vi "Check Loop Error.vi"(9 "Ignore Errors":i32[](array[numeric]) caption="忽略错误", 10 "error to process":errorcluster caption="待处理的错误", 11 "Message Queue":refnum<queue> caption="消息队列") -> (2 "Enqueued Error?":bool caption="错误入队列？", 3 "dup Message Queue":refnum<queue> caption="消息队列副本")   [LabVIEW 2013]
doc: "检查“处理的错误”，查看代码值是否与“忽略错误”数组中的任意值相匹配。如果是，则忽略。如果否，发送包含错误数据的错误信息至消息处理循环，以进行深入处理。"
uses:
  Message Queue/Message Cluster.ctl
  Message Queue/Enqueue Message (Single).vi
  Message Queue/Message Queue.lvlib
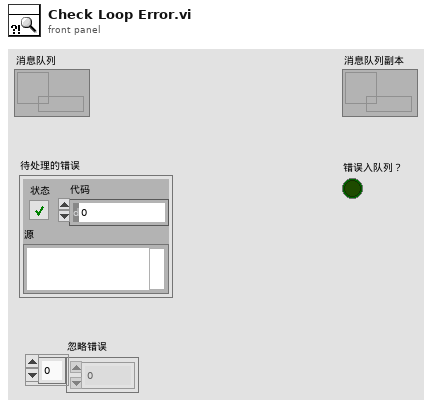
[diagram p1: front panel]
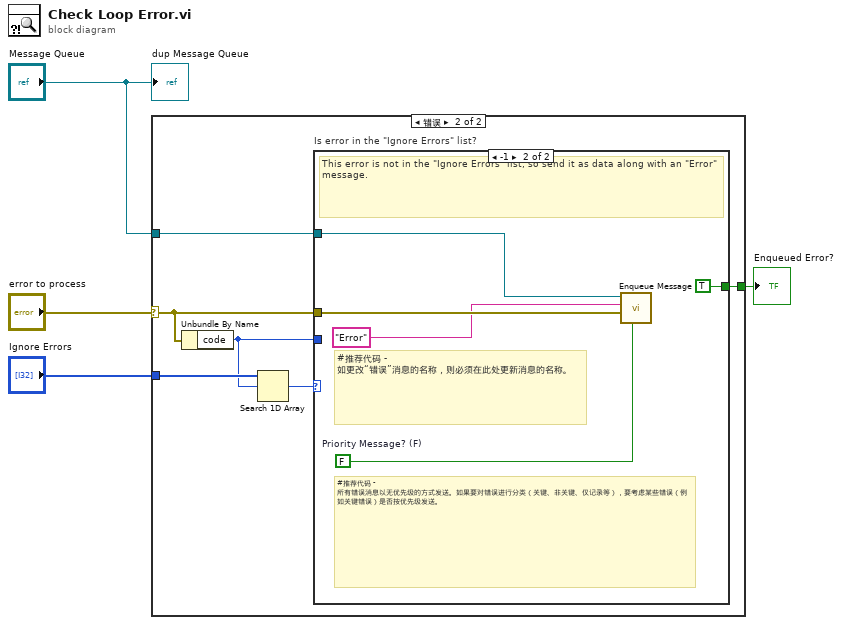
[diagram p0: block diagram]
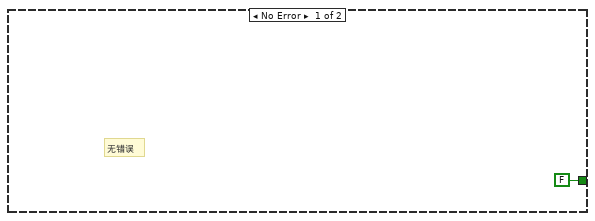
[diagram p2: hidden frame]
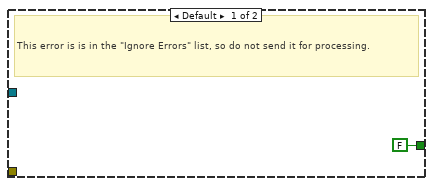
[diagram p3: hidden frame]
diagram:
  n1 = case shown="错误" "error to process" {
    selector: "error to process" -> [_ w7]
    tunnel: "Ignore Errors" -> [_ w11]
    tunnel: "Message Queue" -> [_ w9]
    tunnel: [FALSE ("Enqueued Error?") w6] -> w1
    frame No Error {
      # "无错误"
    }
    frame Error {
      n2 = Unbundle By Name(w7) -> ("code"=w8:i32)
      n3 = Search 1D Array(1D array=w11, element=w8) -> (index of element=w10:i32)  [unwired: 1 in]
      n4 = case "Is error in the \"Ignore Errors\" list?" shown="-1" w10 {
        tunnel: w9 -> [_ w16]
        tunnel: w8 -> [_ _]
        tunnel: w7 -> [_ w17]
        tunnel: [FALSE ("Enqueued Error?") TRUE ("Enqueued Error?")] -> w6
        frame Default {
          # "This error is is in the \"Ignore Errors\" list, so do not send it for processing."
        }
        frame -1 {
          w14 = FALSE  # Priority Message? (F)
          # "#推荐代码 - 所有错误消息以无优先级的方式发送。如果要对错误进行分类（关键、非关键、仅记录等），要考虑某些错误（例如关键错误）是否按优先级发送。"
          # "#推荐代码 - 如更改“错误”消息的名称，则必须在此处更新消息的名称。"
          # "This error is not in the \"Ignore Errors\" list, so send it as data along with an \"Error\" message."
          n5 = call-poly "Enqueue Message.vi"("Priority Message? (F)"=w14, "Message Data"=w17, "Message"="Error", "Message Queue"=w16) -> ()  [unwired: 6 in, 2 out]
        }
      }
    }
  }
  "Enqueued Error?" <- w1
  "dup Message Queue" <- "Message Queue"
